vi "DeployImage.vi"(8 "error in (no error)":errorcluster, 10 "SysCfgDeployPackageRequest":T4, 11 "service":refnum<class "IcmMessageService.lvclass">) -> (0 "error out":errorcluster)   [LabVIEW 2016]
doc: "Queries for all equipment asset nodes, which means they have operating states."
uses:
  <vilib>/addons/InsightCM/MessageBus/MessageService/IcmMessageService.lvclass
  <vilib>/addons/InsightCM/MessageBus/MessageLibrary/SysCfgDeployer/controls/SysCfgDeployPackageRequestBody.ctl
  <vilib>/addons/InsightCM/MessageBus/Base/controls/KeyValuePair.ctl
  <vilib>/addons/InsightCM/MessageBus/Base/controls/MessageHeader.ctl
  <vilib>/addons/InsightCM/MessageBus/MessageLibrary/SysCfgDeployer/controls/SysCfgDeployPackageResponseBody.ctl
panel:
  out "Body":T1
  out "Header":T2
  out "string":string
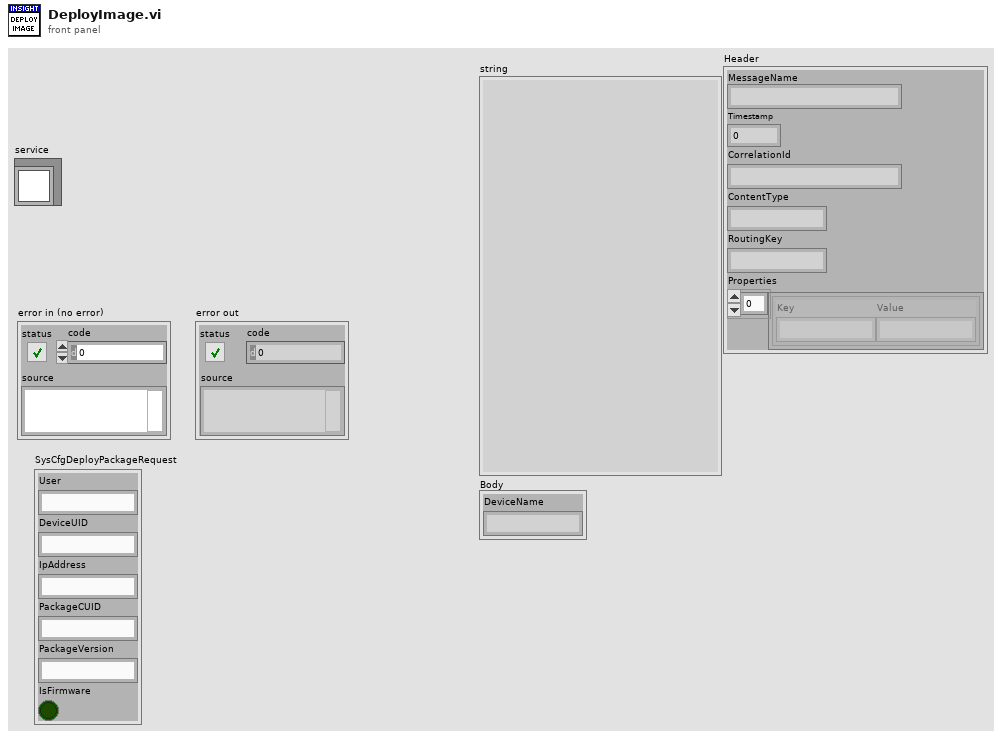
[diagram p1: front panel]
types:
  T1 = typedef "SysCfgDeployPackageResponseBody.ctl" = cluster{"DeviceName":string}
  T2 = typedef "MessageHeader.ctl" = cluster{"MessageName":string, "Timestamp":i64, "CorrelationId":string, "ContentType":string, "RoutingKey":string, "Properties":T3[]}
  T3 = typedef "KeyValuePair.ctl" = cluster{"Key":string, "Value":string}
  T4 = typedef "SysCfgDeployPackageRequestBody.ctl" = cluster{"User":string, "DeviceUID":string, "IpAddress":string, "PackageCUID":string, "PackageVersion":string, "IsFirmware":bool}
  T5 = typedef "Message.ctl" = cluster{"Header":T2, "Body":u8[]}
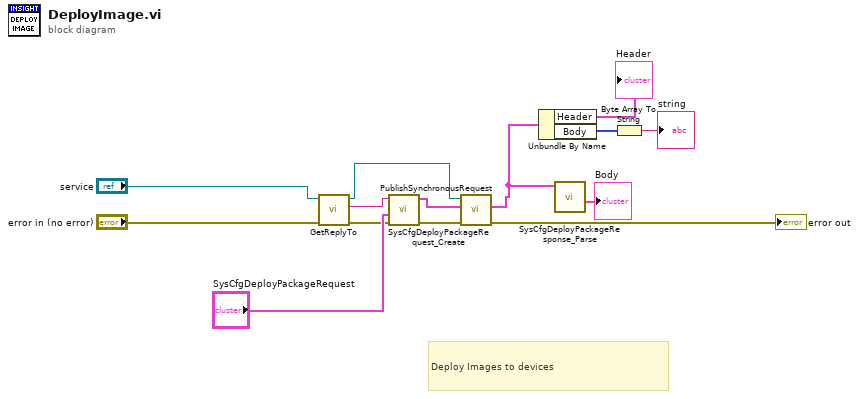
[diagram p0: block diagram]
diagram:
  # "Deploy Images to devices"
  n1 = call <vilib>:"GetReplyTo.vi"("error in (no error)"="error in (no error)", "service in"="service") -> ("error out"=w10:errorcluster, "reply to"=w9:string, "service out"=w12:refnum<class "IcmMessageService.lvclass">)  [unwired: 7 in]
  n2 = call <vilib>:"SysCfgDeployPackageRequest_Create.vi"("error in (no error)"=w10, "SysCfgDeployPackageRequest"="SysCfgDeployPackageRequest", "ReplyTo"=w9) -> ("error out"=w8:errorcluster, "Message"=w7:T5)  [unwired: 7 in]
  n3 = call <vilib>:"PublishSynchronousRequest.vi"("error in (no error)"=w8, "request"=w7, "service in"=w12) -> ("error out"=→"error out":errorcluster, "response"=w2:T5)  [unwired: 6 in, 1 out]
  n4 = Unbundle By Name(w2) -> ("Header"=→"Header":T2, "Body"=w6:u8[])
  n5 = call <vilib>:"SysCfgDeployPackageResponse_Parse.vi"("Message"=w2) -> ("Body"=→"Body":T1)  [unwired: 7 in, 3 out]
  n6 = Byte Array To String(unsigned byte array=w6) -> (string=→"string":string)
